vi "sub_DTMF_Decoder.vi"(8 "SNRdB":dbl, 11 "signal":dbl[](array[numeric])) -> (3 "digits":string)   [LabVIEW 2011]
uses:
  <vilib>/imath/engines/lvmath/Plug In/_Char/NIMS_CH_character datatype.ctl
  <vilib>/imath/engines/lvmath2/RunTimeEngine/ErrorHandling/NIMS_Finalize Error.vi
  <vilib>/imath/engines/lvmath2/RunTimeEngine/RunTimeType/NIMS_RunTimeType_From StrictType (excl LVString).vi
  <instcachedir>/0/NIMS_RunTimeType_From StrictType (excl LVString)_46AE8B54A11948F0BCCEB8091EE7AA4C.lvgen/NIMS_RunTimeType_From StrictType (excl LVString)_46AE8B54A11948F0BCCEB8091EE7AA4C_025.vi
  <vilib>/imath/engines/lvmath2/RunTimeEngine/RunTimeType/NIMS_RunTimeType_Get Case Value.vi
  <vilib>/imath/engines/lvmath2/RunTimeEngine/NodeEndStatement/NIMS_NodeEndStatement_Output.vi
  <instcachedir>/0/NIMS_NodeEndStatement_Output_53EC0D466D134D7ABD903AC30B43404B.lvgen/NIMS_NodeEndStatement_Output_53EC0D466D134D7ABD903AC30B43404B_007.vi
  <vilib>/imath/engines/lvmath2/RunTimeEngine/BuiltInFunctions/filter/NIMS_filter(GV,GV,GV,GV,Str).vi
  <instcachedir>/0/NIMS_filter(GV,GV,GV,GV,Str)_23F9F1BD357242CFB8A4C1E6AAEF1E0F.lvgen/NIMS_filter(GV,GV,GV,GV,Str)_23F9F1BD357242CFB8A4C1E6AAEF1E0F_000.vi
  <vilib>/imathl/engines/lvmath/Functions/Error Handling/Create Error.vi
  <vilib>/imath/engines/lvmath2/RunTimeEngine/BuiltInFunctions/round/NIMS_round(DBL-S).vi
  <vilib>/imath/engines/lvmath2/RunTimeEngine/BuiltInFunctions/round/NIMS_round(DBL-V).vi
  <vilib>/imath/engines/lvmath2/RunTimeEngine/BuiltInFunctions/length/NIMS_length(GV).vi
  <instcachedir>/0/NIMS_length(GV)_08A3D13377FD4E4B96F5795FBF3698FA.lvgen/NIMS_length(GV)_08A3D13377FD4E4B96F5795FBF3698FA_000.vi
  <vilib>/imath/engines/lvmath2/RunTimeEngine/BuiltInFunctions/zeros/NIMS_M=zeros(I32,I32).vi
  <vilib>/imath/engines/lvmath2/RunTimeEngine/RangeToken/NIMS_Range_R2 - Float.vi
  <instcachedir>/0/NIMS_Range_R2 - Float_C1282E71A4144327AAA2CE46E2A27C60.lvgen/NIMS_Range_R2 - Float_C1282E71A4144327AAA2CE46E2A27C60_000.vi
  <vilib>/imath/engines/lvmath2/RunTimeEngine/CommandStatement/MC_CommandStatement_break.vi
  <vilib>/imath/engines/lvmath2/RunTimeEngine/RangeToken/NIMS_Range.vi
  <instcachedir>/0/NIMS_Range_0B7635FB69F84E19AA68E7FF959DF37C.lvgen/NIMS_Range_0B7635FB69F84E19AA68E7FF959DF37C_001.vi
  <vilib>/imath/engines/lvmath2/RunTimeEngine/VariableToken/Read/NIMS_Get Elements - RV(_) - Check(_).vi
  <instcachedir>/0/NIMS_Get Elements - RV(_) - Check(_)_95E78A4FFA0646428F3543E57837F638.lvgen/NIMS_Get Elements - RV(_) - Check(_)_95E78A4FFA0646428F3543E57837F638_001.vi
  <vilib>/imath/engines/lvmath2/RunTimeEngine/BuiltInFunctions/zeros/NIMS_V=zeros(I32,I32).vi
  <vilib>/imath/engines/lvmath2/RunTimeEngine/ErrorHandling/NIMS_Create Error From Enums.vi
  <vilib>/imath/engines/lvmath2/RunTimeEngine/ReplaceToken/NIMS_Replace - Check(_) Row.vi
  <instcachedir>/0/NIMS_Replace - Check(_) Row_E0D5D7FCFC594C9EB27A53B050DE844E.lvgen/NIMS_Replace - Check(_) Row_E0D5D7FCFC594C9EB27A53B050DE844E_001.vi
  <vilib>/imath/engines/lvmath2/RunTimeEngine/RangeToken/NIMS_Range_R2.vi
  <vilib>/imath/engines/lvmath2/RunTimeEngine/VariableToken/Read/NIMS_Get Elements - RV(_) - Check.vi
  <instcachedir>/0/NIMS_Get Elements - RV(_) - Check_B511B9D8E05044FE80F9F088FE24B20C.lvgen/NIMS_Get Elements - RV(_) - Check_B511B9D8E05044FE80F9F088FE24B20C_001.vi
  <vilib>/imath/engines/lvmath2/RunTimeEngine/BuiltInFunctions/goertzel/NIMS_goertzel(GV, I32V).vi
  <instcachedir>/0/NIMS_goertzel(GV, I32V)_044EB06A74B64590A53D4838DA4AC1A9.lvgen/NIMS_goertzel(GV, I32V)_044EB06A74B64590A53D4838DA4AC1A9_001.vi
  <vilib>/imath/engines/lvmath2/RunTimeEngine/ReplaceToken/NIMS_Replace - Size Check M(_,$)=VorM.vi
  <instcachedir>/0/NIMS_Replace - Size Check M(_,$)=VorM_E9325078D1244F22AE546E08DE44A10D.lvgen/NIMS_Replace - Size Check M(_,$)=VorM_E9325078D1244F22AE546E08DE44A10D_011.vi
  <vilib>/imath/engines/lvmath2/RunTimeEngine/ReplaceToken/NIMS_Replace - Assignment Check M(_,$)=VorM.vi
  <instcachedir>/0/NIMS_Replace - Assignment Check M(_,$)=VorM_172B853FB74644F4A2D334A88A052971.lvgen/NIMS_Replace - Assignment Check M(_,$)=VorM_172B853FB74644F4A2D334A88A052971_011.vi
  <vilib>/imath/engines/lvmath2/RunTimeEngine/BuiltInFunctions/abs/NIMS_abs(signed).vi
  <instcachedir>/0/NIMS_abs(signed)_C4FCB8E6058B49B797C7C8D53CA5F6EC.lvgen/NIMS_abs(signed)_C4FCB8E6058B49B797C7C8D53CA5F6EC_003.vi
  <vilib>/imath/engines/lvmath2/RunTimeEngine/BuiltInFunctions/rem/NIMS_rem_no checks.vi
  <instcachedir>/0/NIMS_rem_no checks_8A14A2E4DF484AE391F841C42148F124.lvgen/NIMS_rem_no checks_8A14A2E4DF484AE391F841C42148F124_008.vi
  <vilib>/imath/engines/lvmath2/RunTimeEngine/ReplaceToken/NIMS_Replace - Check Linear.vi
  <instcachedir>/0/NIMS_Replace - Check Linear_276AD648BD064726893CCF9ED6E2A728.lvgen/NIMS_Replace - Check Linear_276AD648BD064726893CCF9ED6E2A728_009.vi
  <vilib>/imath/engines/lvmath2/RunTimeEngine/VariableToken/Read/NIMS_Get Elements - SorM(_) - Check.vi
  <instcachedir>/0/NIMS_Get Elements - SorM(_) - Check_6C920A4996D9400D8D9F035318A663F0.lvgen/NIMS_Get Elements - SorM(_) - Check_6C920A4996D9400D8D9F035318A663F0_001.vi
  <vilib>/imath/engines/lvmath2/RunTimeEngine/ReplaceToken/NIMS_Replace - Size Check _(_)=VorM.vi
  <instcachedir>/0/NIMS_Replace - Size Check _(_)=VorM_C85DCC3888F14C5FACDCACC8CAF67F25.lvgen/NIMS_Replace - Size Check _(_)=VorM_C85DCC3888F14C5FACDCACC8CAF67F25_012.vi
  <vilib>/imath/engines/lvmath2/RunTimeEngine/ReplaceToken/NIMS_Replace - Assignment Check _(_)=VorM.vi
  <instcachedir>/0/NIMS_Replace - Assignment Check _(_)=VorM_486412C526DE41D4B9BEEA980C633181.lvgen/NIMS_Replace - Assignment Check _(_)=VorM_486412C526DE41D4B9BEEA980C633181_012.vi
  <vilib>/imath/engines/lvmath2/RunTimeEngine/BuiltInFunctions/mean/NIMS_RCol=mean(RM,I32).vi
  <vilib>/imath/engines/lvmath2/RunTimeEngine/BuiltInFunctions/max/3 inputs/NIMS_[RCol, Row]=max(RM,M,I32).vi
  <instcachedir>/0/NIMS_[RCol, Row]=max(RM,M,I32)_01E1DA57CF234719B1D4D5BC514486FB.lvgen/NIMS_[RCol, Row]=max(RM,M,I32)_01E1DA57CF234719B1D4D5BC514486FB_000.vi
  <vilib>/imath/engines/lvmath2/RunTimeEngine/ArithmeticOperatorToken/NIMS_ArithmeticOperator_rightdiv.vi
  <instcachedir>/0/NIMS_ArithmeticOperator_rightdiv_85C5B8074732470A99000A2C3876C445.lvgen/NIMS_ArithmeticOperator_rightdiv_85C5B8074732470A99000A2C3876C445_000.vi
  <vilib>/imath/engines/lvmath2/RunTimeEngine/BuiltInFunctions/ones/NIMS_V=ones(I32,I32).vi
  <vilib>/imath/engines/lvmath2/RunTimeEngine/VariableToken/Read/NIMS_Get Elements - CV(_,_) - Check(_) - NoCheck.vi
  <instcachedir>/0/NIMS_Get Elements - CV(_,_) - Check(_) - NoCheck_EF626B273E124C0AB978B8F37981BA8F.lvgen/NIMS_Get Elements - CV(_,_) - Check(_) - NoCheck_EF626B273E124C0AB978B8F37981BA8F_000.vi
  <instcachedir>/0/NIMS_Get Elements - CV(_,_) - Check(_) - NoCheck_EF626B273E124C0AB978B8F37981BA8F.lvgen/NIMS_Get Elements - CV(_,_) - Check(_) - NoCheck_EF626B273E124C0AB978B8F37981BA8F_001.vi
  <vilib>/imath/engines/lvmath2/RunTimeEngine/VariableToken/Read/NIMS_Get Elements - SorM(_,_) - Check(_) - Check.vi
  <instcachedir>/0/NIMS_Get Elements - SorM(_,_) - Check(_) - Check_BBF62745DD224AEFA8FD4D9A9401DF8A.lvgen/NIMS_Get Elements - SorM(_,_) - Check(_) - Check_BBF62745DD224AEFA8FD4D9A9401DF8A_000.vi
  <instcachedir>/0/NIMS_Replace - Check(_) Row_E0D5D7FCFC594C9EB27A53B050DE844E.lvgen/NIMS_Replace - Check(_) Row_E0D5D7FCFC594C9EB27A53B050DE844E_009.vi
  <vilib>/imath/engines/lvmath2/RunTimeEngine/ReplaceToken/NIMS_Replace - Check Column.vi
  <instcachedir>/0/NIMS_Replace - Check Column_7A54AC4688FE427CA8C7A22E1199AA47.lvgen/NIMS_Replace - Check Column_7A54AC4688FE427CA8C7A22E1199AA47_007.vi
  <vilib>/imath/engines/lvmath2/RunTimeEngine/ReplaceToken/NIMS_Replace - Size Check M(_,_)=S.vi
  <instcachedir>/0/NIMS_Replace - Size Check M(_,_)=S_7A52A38CE0894443836533BCD5872384.lvgen/NIMS_Replace - Size Check M(_,_)=S_7A52A38CE0894443836533BCD5872384_002.vi
  <vilib>/imath/engines/lvmath2/RunTimeEngine/ReplaceToken/NIMS_Replace - M(S,S)=S.vi
  <instcachedir>/0/NIMS_Replace - M(S,S)=S_4F64D24AC6B044CE86336B8F95ECD677.lvgen/NIMS_Replace - M(S,S)=S_4F64D24AC6B044CE86336B8F95ECD677_002.vi
  <vilib>/imath/engines/lvmath2/RunTimeEngine/VariableToken/Read/NIMS_Get Elements - SorM(_) - Check(_).vi
  <instcachedir>/0/NIMS_Get Elements - SorM(_) - Check(_)_561A7B7910804DA3BBA41B7F4E44AAB4.lvgen/NIMS_Get Elements - SorM(_) - Check(_)_561A7B7910804DA3BBA41B7F4E44AAB4_008.vi
  <vilib>/imath/engines/lvmath2/RunTimeEngine/RowToken/NIMS_RowToken_M_SorRV.vi
  <instcachedir>/0/NIMS_RowToken_M_SorRV_7D706DDE498144F993BC9D4030E937C1.lvgen/NIMS_RowToken_M_SorRV_7D706DDE498144F993BC9D4030E937C1_001.vi
  <instcachedir>/0/NIMS_RunTimeType_From StrictType (excl LVString)_46AE8B54A11948F0BCCEB8091EE7AA4C.lvgen/NIMS_RunTimeType_From StrictType (excl LVString)_46AE8B54A11948F0BCCEB8091EE7AA4C_006.vi
  C:/Users/Daniel/Documents/LabVIEW Data/MathScriptVIs/MCStatic_285220864_937560ddfe5eb705a28285b480da4e66.vi
  <instcachedir>/0/MCStatic_285220864_937560ddfe5eb705a28285b480da4e66_88E6CF4FF5214472B23233C46A7170A2.lvgen/MCStatic_285220864_937560ddfe5eb705a28285b480da4e66_88E6CF4FF5214472B23233C46A7170A2_000.vi
  <vilib>/imath/engines/lvmath2/RunTimeEngine/VariableToken/Read/NIMS_Get Elements - SorM(_,_) - Check - Check.vi
  <instcachedir>/0/NIMS_Get Elements - SorM(_,_) - Check - Check_DA1E252EAB634D989357E7C72E8137F5.lvgen/NIMS_Get Elements - SorM(_,_) - Check - Check_DA1E252EAB634D989357E7C72E8137F5_006.vi
  <vilib>/imath/engines/lvmath2/RunTimeEngine/RunTimeType/NIMS_RunTimeType_To Numeric.vi
  <instcachedir>/0/NIMS_RunTimeType_To Numeric_23D8CB4491074484AE5B88877770AD36.lvgen/NIMS_RunTimeType_To Numeric_23D8CB4491074484AE5B88877770AD36_005.vi
  <vilib>/imath/engines/lvmath/Plug In/_Char/NIMS_CH_U8 2D to Character 2D.vi
  <instcachedir>/0/NIMS_RowToken_M_SorRV_7D706DDE498144F993BC9D4030E937C1.lvgen/NIMS_RowToken_M_SorRV_7D706DDE498144F993BC9D4030E937C1_003.vi
  <vilib>/imath/engines/lvmath/Plug In/_Char/RunTimeType/NIMS_CH_RunTimeType_To Character 1D.vi
  <instcachedir>/0/MCStatic_285220864_937560ddfe5eb705a28285b480da4e66_88E6CF4FF5214472B23233C46A7170A2.lvgen/MCStatic_285220864_937560ddfe5eb705a28285b480da4e66_88E6CF4FF5214472B23233C46A7170A2_001.vi
  <vilib>/imath/engines/lvmath2/RunTimeEngine/NodeEndStatement/NIMS_NodeEndStatement_Get Vector.vi
  <instcachedir>/0/NIMS_NodeEndStatement_Get Vector_50E2F48DC826428EA11CD85545CBACBE.lvgen/NIMS_NodeEndStatement_Get Vector_50E2F48DC826428EA11CD85545CBACBE_003.vi
  <vilib>/imath/engines/lvmath/Plug In/_Char/NIMS_CH_U8 1D to Character 1D.vi
  <vilib>/imath/engines/lvmath/Plug In/_Char/NIMS_CH_Character RV to String.vi
  mode.m
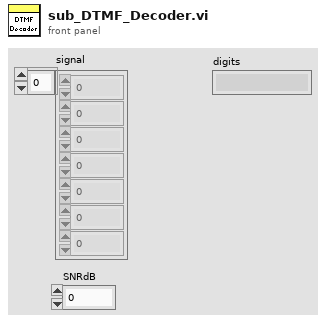
[diagram p1: front panel]
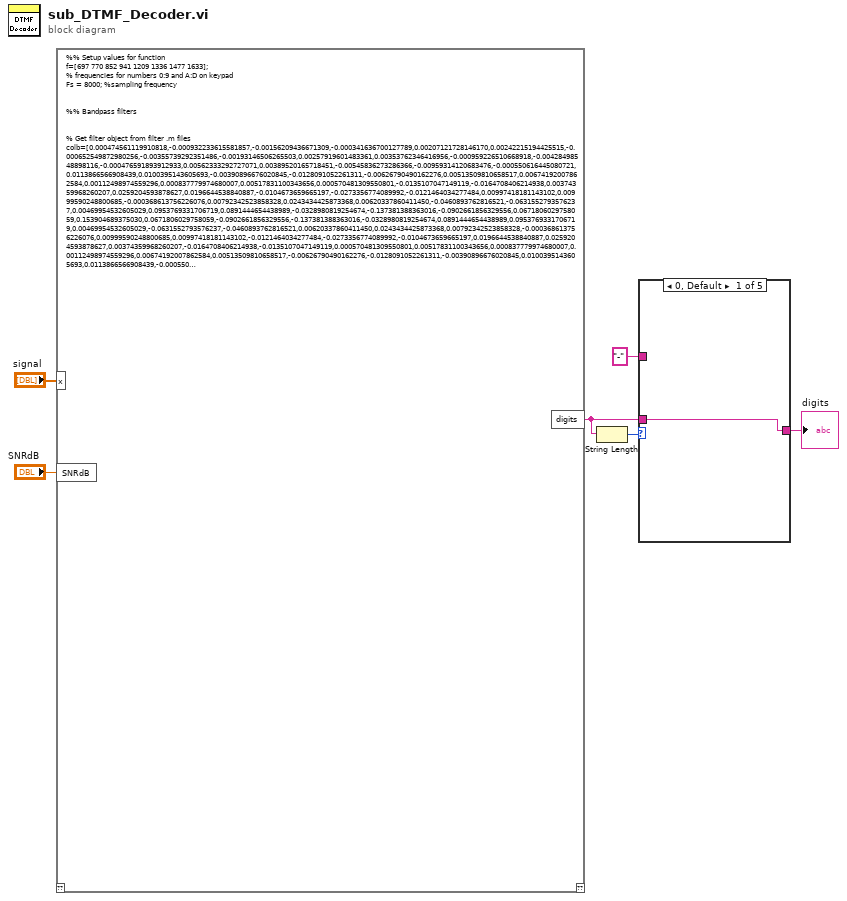
[diagram p0: block diagram]
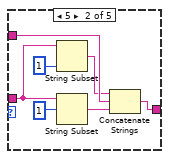
[diagram p2: hidden frame]
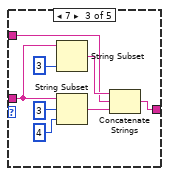
[diagram p3: hidden frame]
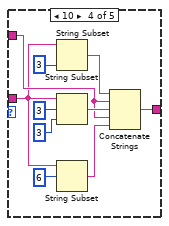
[diagram p4: hidden frame]
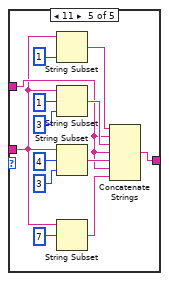
[diagram p5: hidden frame]
diagram:
  n1 = mathscript code="%% Setup values for function\nf=[697 770 852 941 1209 1336 1477 1633];\n% frequencies for numbers 0:9 and A:D on keypad\nFs = 8000; %sampling frequency\n\n\n%% Bandpass filters\n\n\n% Get filter object from filter .m files\ncolb=[0.000474561119910818,-0.000932233615581857,-0.00156209436671309,-0.000341636700127789,0.00207121728146170,0.00242215194425515,-0.000652549872980256,-0.00355739292351486,-0.00193146506265503,0.00257919601483361,0.00353762346416956,-0.000959226510668918,-0.00428498548898116,-0.000476591893912933,0.00562333292727071,0.00389520165718451,-0.00545836273286366,-0.00959314120683476,-0.000550616445080721,0.0113866566908439,0.0100395143605693,-0.00390896676020845,-0.0128091052261311,-0.00626790490162276,0.00513509810658517,0.00674192007862584,0.00112498974559296,0.000837779974680007,0.00517831100343656,0.000570481309550801,-0.0135107047149119,-0.0164708406214938,0.00374359968260207,0.0259204593878627,0.0196644538840887,-0.0104673659665197,-0.0273356774089992,-0.0121464034277484,0.00997418181143102,0.00999590248800685,-0.000368613756226076,0.00792342523858328,0.0243434425873368,0.00620337860411450,-0.0460893762816521,-0.0631552793576237,0.00469954532605029,0.0953769331706719,0.0891444654438989,-0.0328980819254674,-0.137381388363016,-0.0902661856329556,0.0671806029758059,0.153904689375030,0.0671806029758059,-0.0902661856329556,-0.137381388363016,-0.0328980819254674,0.0891444654438989,0.0953769331706719,0.00469954532605029,-0.0631552793576237,-0.0460893762816521,0.00620337860411450,0.0243434425873368,0.00792342523858328,-0.000368613756226076,0.00999590248800685,0.00997418181143102,-0.0121464034277484,-0.0273356774089992,-0.0104673659665197,0.0196644538840887,0.0259204593878627,0.00374359968260207,-0.0164708406214938,-0.0135107047149119,0.000570481309550801,0.00517831100343656,0.000837779974680007,0.00112498974559296,0.00674192007862584,0.00513509810658517,-0.00626790490162276,-0.0128091052261311,-0.00390896676020845,0.0100395143605693,0.0113866566908439,-0.000550616445080721,-0.00959314120683476,-0.00545836273286366,0.00389520165718451,0.00562333292727071,-0.000476591893912933,-0.00428498548898116,-0.000959226510668918,0.00353762346416956,0.00257919601483361,-0.00193146506265503,-0.00355739292351486,-0.000652549872980256,0.00242215194425515,0.00207121728146170,-0.000341636700127789,-0.00156209436671309,-0.000932233615581857,0.000474561119910818;];\nrowb=[0.000945787956669407,0.000372595379142179,-0.000414658405181117,-0.00174339905881631,-0.00300754607323483,-0.00327061158896733,-0.00174459191175499,0.00159938897810475,0.00566028615103016,0.00843636687026031,0.00792463567790728,0.00333222891486382,-0.00409318139955560,-0.0112479047364019,-0.0145206320853615,-0.0117269697295376,-0.00355785298609024,0.00643958109070302,0.0135611171174945,0.0145156384247386,0.00937469861323721,0.00160859847386289,-0.00402112306666083,-0.00455527848099008,-0.000966673450745421,0.00224520237542859,7.44279609591604e-05,-0.00904476478078409,-0.0209794496468590,-0.0272426377709717,-0.0197855880924097,0.00322917730447459,0.0342786326660773,0.0585130394018876,0.0607697679939461,0.0342512998693288,-0.0139683348058471,-0.0642865184648740,-0.0929752288069270,-0.0838738927157436,-0.0373832358356305,0.0282866095775546,0.0848287424289370,0.107020087276661,0.0848287424289370,0.0282866095775546,-0.0373832358356305,-0.0838738927157436,-0.0929752288069270,-0.0642865184648740,-0.0139683348058471,0.0342512998693288,0.0607697679939461,0.0585130394018876,0.0342786326660773,0.00322917730447459,-0.0197855880924097,-0.0272426377709717,-0.0209794496468590,-0.00904476478078409,7.44279609591604e-05,0.00224520237542859,-0.000966673450745421,-0.00455527848099008,-0.00402112306666083,0.00160859847386289,0.00937469861323721,0.0145156384247386,0.0135611171174945,0.00643958109070302,-0.00355785298609024,-0.0117269697295376,-0.0145206320853615,-0.0112479047364019,-0.00409318139955560,0.00333222891486382,0.00792463567790728,0.00843636687026031,0.00566028615103016,0.00159938897810475,-0.00174459191175499,-0.00327061158896733,-0.00300754607323483,-0.00174339905881631,-0.000414658405181117,0.000372595379142179,0.000945787956669407;];\n\n% Apply column and row signal to signal\nrowFilt=filter(rowb,1,x);\ncolFilt=filter(colb,1,x);\n\n\n%% Create Windows\n% Desired frequency resolution 73 Hz thus with a rectangular window the\n% peak to null resolution is 1/T. To get T >=13.7 ms we need M=110. M=106\n% gives 13.3 ms and gives two full windows in 40 ms.\nL=106;\n\n% Time to index converstions\nt_10ms=round(Fs/L*0.010);\nt_23ms=round(Fs/L*0.023);\nt_40ms=round(Fs/L*0.040);\n\n\n%% Goertzel DFT\nN_fundamental = 205; %Number of points for DFT of fundamentals\nN_harmonics = 201; %Number of points for DFT of harmonics\n\n% Indices of the DFT for the frequencies f \nfreq_indices = round(f/Fs*N_fundamental)+1;\nharmonic_indicies = round(f*2/Fs*N_harmonics)+1;\n\n% Calculate number of windows in sample with given window size\nnWindows=floor(length(x)/L)-1;\n\ndft_col=zeros(nWindows,4);\ndft_col_harmonic=zeros(nWindows,4);\ndft_row=zeros(nWindows,4);\ndft_row_harmonic=zeros(nWindows,4);\nfor n=1:nWindows\n    %Compute DFT of fundamentals using Goertzel algorithm\n    padded_col=[colFilt(n*L:(n+1)*L),zeros(1,N_fundamental-L)];\n    padded_row=[rowFilt(n*L:(n+1)*L),zeros(1,N_fundamental-L)];\n    dft_col(n,:) = goertzel(padded_col,freq_indices(5:end));\n    dft_row(n,:) = goertzel(padded_row,freq_indices(1:4));\n    \n    %Compute DFT of harmonics using Goertzel algorithm\n    padded_col_harmonics=[colFilt(n*L:(n+1)*L),zeros(1,N_harmonics-L)];\n    padded_row_harmonics=[rowFilt(n*L:(n+1)*L),zeros(1,N_harmonics-L)];\n    dft_col_harmonic(n,:) = goertzel(padded_col_harmonics,harmonic_indicies(5:end));\n    dft_row_harmonic(n,:) = goertzel(padded_row_harmonics,harmonic_indicies(1:4));\nend\n\n\n%% Calculate Signal Power\n\n% Compute average power\n% Take the magnitude of dft of x and scale the dft so that it is not a \n% function of the window length\n\ncol_power = abs(dft_col)/L; \ncol_harmonic_power = abs(dft_col_harmonic)/L; \nrow_power = abs(dft_row)/L; \nrow_harmonic_power = abs(dft_row_harmonic)/L;\n\n% Take the square of the magnitude of dft of windowed x. \n\ncol_power = col_power.^2; \ncol_harmonic_power = col_harmonic_power.^2;\nrow_power = row_power.^2;\nrow_harmonic_power = row_harmonic_power.^2;\n\n% We multiply mx by 2 to keep the same energy as the symetric dft.\n% The DC component and Nyquist component, if it exists, are unique\n% and should not be multiplied by 2.\n\nif rem(N_fundamental, 2) % odd dft excludes Nyquist point\n  col_power(2:end) = col_power(2:end)*2;\n  col_harmonic_power(2:end) = col_harmonic_power(2:end)*2;\n  row_power(2:end) = row_power(2:end)*2;\n  row_harmonic_power(2:end) = row_harmonic_power(2:end)*2;\nelse\n  col_power(2:end -1) = col_power(2:end -1)*2;\n  col_harmonic_power(2:end-1) = col_harmonic_power(2:end-1)*2;\n  row_power(2:end -1) = row_power(2:end -1)*2;\n  row_harmonic_power(2:end-1) = row_harmonic_power(2:end-1)*2;\nend\n\n\n% Calculate average power for row freqs and column freqs.\navg_col_power = mean(col_power,2); \navg_row_power = mean(row_power,2); \n\n% Calculate max power for row freqs and column freqs.\n[max_col_power,max_col_power_index] = max(col_power,[],2); \n[max_row_power,max_row_power_index] = max(row_power,[],2);\n\n% Calculate ratio of max power to avg power for row freqs and column freqs.\nratio_col_power = max_col_power./avg_col_power;\nratio_row_power = max_row_power./avg_row_power;\n\n%% Logic to determine if it is a key press\npower_ratio_thresh=2;\nharmonic_ratio_thresh=2;\npower_thresh=10e-3;\n\n% Set all guesses to -1 to indicate that a frequency was not detected in\n% that window\ncol_freq_guess=ones(nWindows,1)*-1;\nrow_freq_guess=ones(nWindows,1)*-1;\n\nfor n=1:nWindows\n    ratio_test=ratio_col_power(n,1)>power_ratio_thresh &&...\n            ratio_row_power(n,1)>power_ratio_thresh;\n        \n    threshold_test=max_col_power(n,1)>power_thresh &&...\n            max_row_power(n,1)>power_thresh;\n        \n    if (ratio_test && threshold_test)\n        % Calculate ratio of 2nd harmonic to fundamental to check for voice\n        col_harmonic_ratio=col_harmonic_power(n,max_col_power_index(n,1))/col_power(n,max_col_power_index(n,1));\n        row_harmonic_ratio=row_harmonic_power(n,max_row_power_index(n,1))/row_power(n,max_row_power_index(n,1));\n        if (col_harmonic_ratio<harmonic_ratio_thresh && row_harmonic_ratio<harmonic_ratio_thresh)\n            col_freq_guess(n,1)=max_col_power_index(n,1);\n            row_freq_guess(n,1)=max_row_power_index(n,1);\n        end\n    end\nend\n\n%% Key Press Logic\n\nkeys = ['1','2','3','A'; \n        '4','5','6','B';\n        '7','8','9','C';\n        '*','0','#','D']; \n\n% Initialize counters\nsignal_counter=0;  \nsilence_counter=0;\ndigits=[];\ncol_guess=[];\nrow_guess=[];\nfor n=1:nWindows\n    \n    % Test if there is a pair of freqs\n    isKey=col_freq_guess(n)>0 && row_freq_guess(n)>0;\n    \n    % If a key is pressed, test duration rules\n    switch isKey\n        case true\n            col_guess=[col_guess col_freq_guess(n)]; %Index of guessed col\n            row_guess=[row_guess row_freq_guess(n)]; %Index of guessed row\n            % Check if previous signal was interrupted for >10ms.\n            if(silence_counter>t_10ms)  \n                % Check if previous signal was at least 23ms\n                if(signal_counter>t_23ms)\n                    % Find the mode of the previous guesses to account for\n                    % any anomalous frequency pairs\n                    key_col=mode(col_guess);\n                    key_row=mode(row_guess);\n                    % Add digit to digits string\n                    digits=[digits keys(key_row,key_col)];\n                end\n                signal_counter=1; % Start new signal counter\n                silence_counter=0; % Reset silence_counter\n                col_guess=[]; % Reset column guesses\n                row_guess=[]; % Reset row guesses\n            else\n                % Since interruption was <10ms, assume signal is continuing\n                signal_counter=signal_counter+1; % Increment signal counter\n                silence_counter=0; % Reset silence_counter\n            end\n        case false\n            silence_counter=silence_counter+1; % Increment silence counter\n    end\nend\n\n% Check if an additional digit was registers if last window contained a\n% signal\nif(signal_counter>t_23ms)\n    key_col=mode(col_guess);\n    key_row=mode(row_guess);\n    digits=[digits keys(key_row,key_col)];\nend"("x"="signal", "SNRdB"="SNRdB") -> ("digits"=w3:string)  [unwired: 1 in, 1 out]
  n2 = String Length(string=w3) -> (length=w4:i32)
  n3 = case shown="0, Default" w4 {
    tunnel: [w7 w13 w17 w27 w38] -> w2
    tunnel: w3 -> [w7 w10 w15 w23 w34]
    tunnel: "-" -> [_ w12 w16 w24 w36]
    frame 0, Default {
    }
    frame 5 {
      n4 = String Subset(string=w10, length (rest)=1 ("length (rest)")) -> (substring=w11:string)  [unwired: 1 in]
      n5 = String Subset(string=w10, offset (0)=1) -> (substring=w9:string)  [unwired: 1 in]
      n6 = Concatenate Strings(w11, w12, w9) -> (w13:string)
    }
    frame 7 {
      n7 = String Subset(string=w15, length (rest)=3 ("length (rest)")) -> (substring=w21:string)  [unwired: 1 in]
      n8 = String Subset(string=w15, offset (0)=3, length (rest)=4 ("length (rest)")) -> (substring=w20:string)
      n9 = Concatenate Strings(w21, w16, w20) -> (w17:string)
    }
    frame 10 {
      n10 = String Subset(string=w23, length (rest)=3 ("length (rest)")) -> (substring=w31:string)  [unwired: 1 in]
      n11 = String Subset(string=w23, offset (0)=3, length (rest)=3 ("length (rest)")) -> (substring=w30:string)
      n12 = String Subset(string=w23, offset (0)=6) -> (substring=w25:string)  [unwired: 1 in]
      n13 = Concatenate Strings(w31, w24, w30, w24, w25) -> (w27:string)
    }
    frame 11 {
      n14 = String Subset(string=w34, length (rest)=1 ("length (rest)")) -> (substring=w35:string)  [unwired: 1 in]
      n15 = String Subset(string=w34, offset (0)=1, length (rest)=3 ("length (rest)")) -> (substring=w44:string)
      n16 = String Subset(string=w34, offset (0)=4, length (rest)=3 ("length (rest)")) -> (substring=w43:string)
      n17 = String Subset(string=w34, offset (0)=7) -> (substring=w39:string)  [unwired: 1 in]
      n18 = Concatenate Strings(w35, w36, w44, w36, w43, w36, w39) -> (w38:string)
    }
  }
  "digits" <- w2
